vi "Untitled 1.vi"() -> ()   [LabVIEW 2014]
uses:
  <vilib>/measure/NI_MABase.lvlib
  <vilib>/DAQmx/configure/timing.llb/DAQmx Timing (Sample Clock).vi
  <vilib>/DAQmx/create/channels.llb/DAQmx Create Channel (AO-Voltage-Basic).vi
  <vilib>/DAQmx/write.llb/DAQmx Write (Analog 1D DBL 1Chan NSamp).vi
panel:
  in  "samples per channel":i32=1000
  in  "White noise seconds":dbl=0.1
  out "White noise":errorcluster
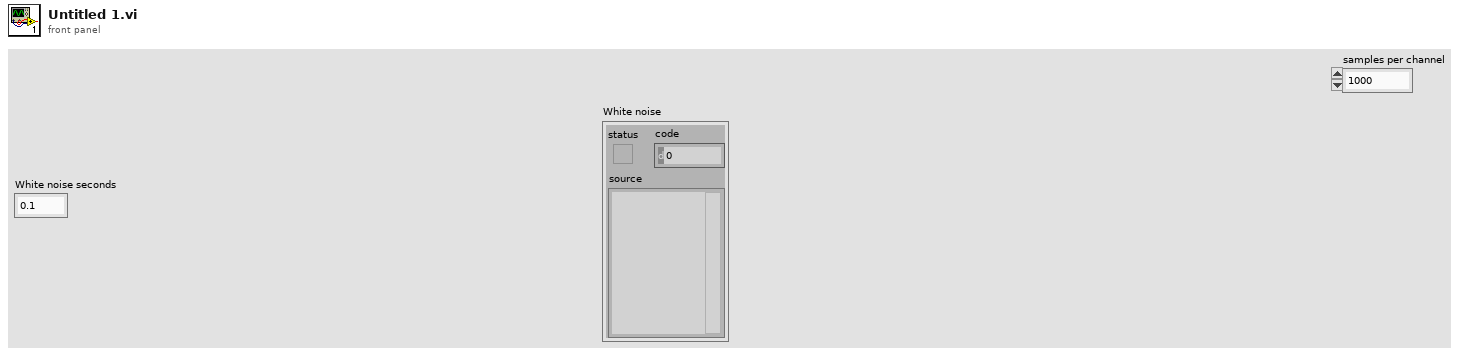
[diagram p1: front panel]
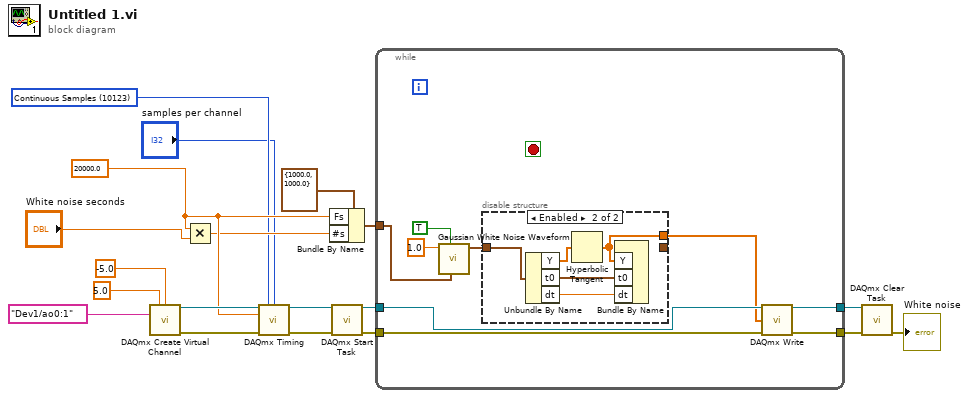
[diagram p0: block diagram]
diagram:
  w2 = 10123 items=["Finite Samples"=10178, "Continuous Samples"=10123, "Hardware Timed Single Point"=12522] ("sample mode")
  w4 = 20000.0 ("rate")
  n1 = call-poly <vilib>:"DAQmx Create Virtual Channel.vi"("maximum value"=5.0, "minimum value"=-5.0, "physical channels"=tag "Dev1/ao0:1") -> ("task out"=w8:refnum<k21>, "error out"=w9:errorcluster)  [unwired: 11 in]
  n2 = Multiply(x=w4, y="White noise seconds") -> (x*y=w3:dbl)
  n3 = call-poly <vilib>:"DAQmx Timing.vi"("task/channels in"=w8, "sample mode"=w2, "samples per channel"="samples per channel", "rate"=w4, "error in"=w9) -> ("task out"=w10:refnum<k21>, "error out"=w11:errorcluster)  [unwired: 9 in]
  n4 = Bundle By Name(cluster=cluster{"Fs":dbl, "#s":dbl} {"Fs"=1000.0, "#s"=1000.0} ("sampling info"), "Fs"=w4, "#s"=w3) -> (w7:cluster{"Fs":dbl, "#s":dbl})
  n5 = call <vilib>:"DAQmx Start Task.vi"("task/channels in"=w10, "error in"=w11) -> ("task out"=w15:refnum<k21>, "error out"=w16:errorcluster)  [unwired: 12 in]
  n6 = while {
    tunnel: w16 -> [w27]
    tunnel: w15 -> [w26]
    tunnel: [w24] -> w14
    tunnel: [w25] -> w13
    tunnel: w7 -> [w21]
    stop <- _ stop-if-true
    n7 = call <vilib>:"Gaussian White Noise Waveform.vi"("sampling info"=w21, "reset signal"=TRUE, "standard deviation"=1.0) -> ("signal out"=w22:waveform(dbl))  [unwired: 7 in, 1 out]
    n8 = disable-structure shown="Enabled" {
      disable-tunnel: [w29 _] -> _
      disable-tunnel: w22 -> [w29 w31]
      disable-tunnel: [_ w30] -> w20
      frame Disabled {
      }
      frame Enabled {
        n9 = Unbundle By Name(w31) -> ("Y"=w34:dbl[], "t0"=w33:timestamp, "dt"=w32:dbl)
        n10 = Hyperbolic Tangent(1:w34) -> (0:w30:dbl[])
        n11 = Bundle By Name("Y"=w30, "t0"=w33, "dt"=w32) -> ()  [unwired: 1 in, 1 out]
      }
    }
    n12 = call-poly <vilib>:"DAQmx Write.vi"("task/channels in"=w26, "data"=w20, "error in"=w27) -> ("task out"=w24:refnum<k21>, "error out"=w25:errorcluster)  [unwired: 10 in, 1 out]
  }
  n13 = call <vilib>:"DAQmx Clear Task.vi"("task in"=w14, "error in"=w13) -> ("error out"=→"White noise":errorcluster)  [unwired: 13 in]
